vi "Test Set Row Values Append Numbers.vi"(11 "Test Case In":refnum<class "Test Open Xml.lvclass">) -> (0 "error out":errorcluster, 3 "Test Case Out":refnum<class "Test Open Xml.lvclass">)   [LabVIEW 2020, in "Test Open Xml.lvclass"]
uses:
  Test Open Xml.lvclass
  <vilib>/Astemes/LUnit/Test Case.lvclass
  Source/Open Xml.lvlib
  Source/Cell DataType.ctl
panel:
  out "Numeric":dbl
  # "200 - 3.6sec"
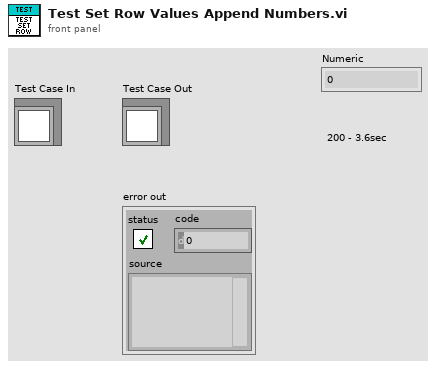
[diagram p1: front panel]
types:
  T1 = typedef "Open Xml.lvlib/Cell DataType.ctl" = enum16{"Void", "Boolean", "Number", "Error", "SharedString", "String", "InlineString", "Date"}
  T2 = cluster{"Number":dbl, "String":string, "Boolean":bool, "Time Stamp":timestamp, "Error":errorcluster}[]
  T3 = cluster{"Number":dbl, "String":string, "Boolean":bool, "Time Stamp":timestamp, "Error":errorcluster}
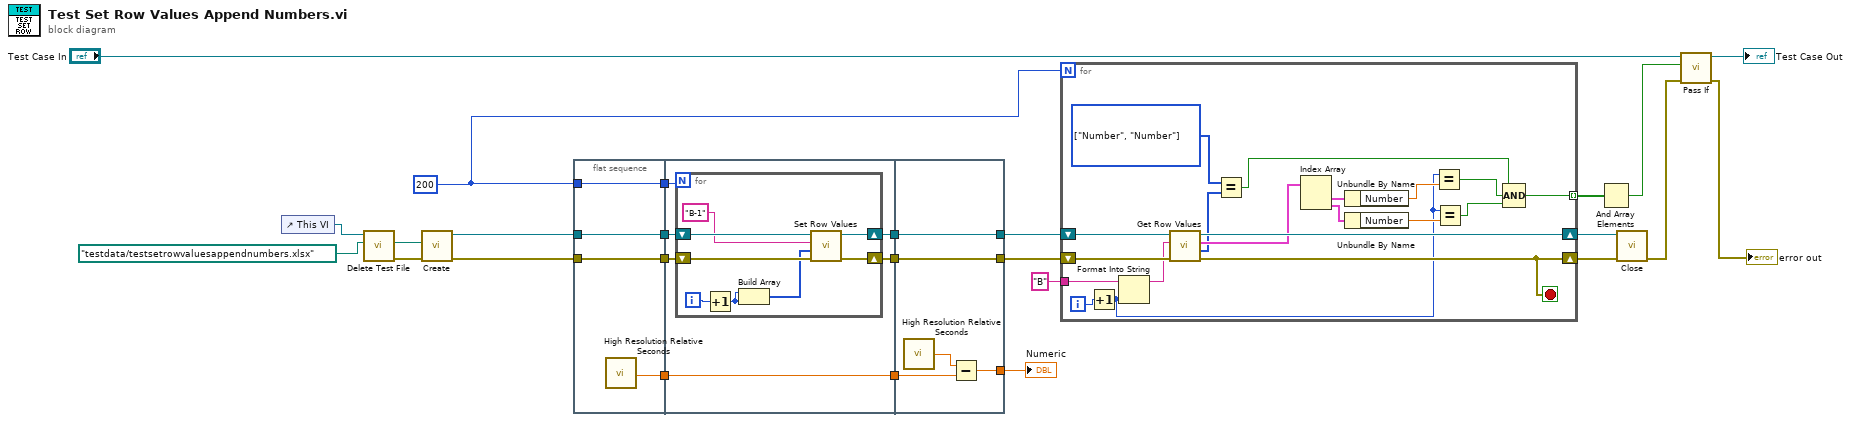
[diagram p0: block diagram]
diagram:
  w11 = 200
  n1 = control-ref of="This VI"() -> (w14:refnum<vi>)
  n2 = call "Delete Test File.vi"("name or relative path"=path "testdata/testsetrowvaluesappendnumbers.xlsx", "VI in"=w14) -> ("error out"=w15:errorcluster, "deleted path"=w12:path)  [unwired: 8 in]
  n3 = call "Create.vi"("error in"=w15, "Path"=w12) -> ("error out"=w22:errorcluster, "SpreadsheetDoc"=w23:refnum<k24>)  [unwired: 8 in]
  n4 = flat-sequence {
    tunnel: w11 -> [w28]
    tunnel: w22 -> [w29]
    tunnel: w23 -> [w30]
    tunnel: [w30] -> w8
    tunnel: [w29] -> w7
    tunnel: [w28] -> w6
    tunnel: [w27] -> w3
    tunnel: w8 -> [w36]
    tunnel: w7 -> [w35]
    tunnel: w6 -> [w32]
    tunnel: [w34] -> w5
    tunnel: [w33] -> w4
    tunnel: w3 -> [w31]
    tunnel: [w31] -> w2
    tunnel: [w48] -> w18
    tunnel: [w49] -> w19
    tunnel: w5 -> [w49]
    tunnel: w4 -> [w48]
    tunnel: w2 -> [w46]
    tunnel: [w45] -> w1
    frame #0 {
      n5 = call <vilib>:"High Resolution Relative Seconds.vi"() -> ("relative seconds"=w27:dbl)
    }
    frame #1 {
      n6 = for {
        N: w32 -> [_]
        shift-right: [w41] -> w33
        shift-left: w36 -> [w44]
        shift-right: [w42] -> w34
        shift-left: w35 -> [w43]
        i -> [w39]
        n7 = Increment(x=w39) -> (x+1=w38:i32)
        n8 = Build Array(w38, w38) -> (w37:i32[])
        n9 = call "Set Row Values.vi"("error in"=w43, "Values"=w37, "Cell Address"="B-1", "SpreadsheetDoc"=w44) -> ("error out"=w42:errorcluster, "SpreadsheetDoc out"=w41:refnum<k24>)  [unwired: 6 in]
      }
    }
    frame #2 {
      n10 = call <vilib>:"High Resolution Relative Seconds.vi"() -> ("relative seconds"=w47:dbl)
      n11 = Subtract(x=w47, y=w46) -> (x-y=w45:dbl)
    }
  }
  n12 = for {
    N: w11 -> [_]
    tunnel: "B" ("Cell Address") -> [w66]
    shift-right: [w51] -> w20
    shift-left: w19 -> [w68]
    shift-right: [w65] -> w16
    shift-left: w18 -> [w67]
    tunnel: [w52] -> w10 mode=indexing
    i -> [w63]
    stop <- w51 stop-if-true
    w62 = T1[] [enum."Number", enum."Number"] items=["Void", "Boolean", "Number", "Error", "SharedString", "String", "InlineString", "Date"] ("x")
    n13 = Increment(x=w63) -> (x+1=w50:i32)
    n14 = Format Into String(initial string=w66, w50) -> (resulting string=w64:string)  [unwired: 2 in, 1 out]
    n15 = call "Get Row Values.vi"("error in"=w68, "Row Address"=w64, "SpreadsheetDoc in"=w67) -> ("error out"=w51:errorcluster, "Types"=w56:T1[], "Cell Values"=w61:T2, "SpreadsheetDoc out"=w65:refnum<k24>)  [unwired: 5 in]
    n16 = Equal?(x=w62, y=w56) -> (x = y?=w53:bool)
    n17 = Index Array(array=w61) -> (element #1=w60:T3, element #2=w59:T3)  [unwired: 2 in]
    n18 = Unbundle By Name(w60) -> ("Number"=w57:dbl)
    n19 = Unbundle By Name(w59) -> ("Number"=w58:dbl)
    n20 = Equal?(x=w50, y=w57) -> (x = y?=w54:bool)
    n21 = Equal?(x=w50, y=w58) -> (x = y?=w55:bool)
    n22 = Compound Arithmetic op=AND(w53, w54, w55) -> (w52:bool)
  }
  n23 = And Array Elements(Boolean array=w10) -> (logical AND=w9:bool)
  n24 = call "Close.vi"("error in"=w20, "SpreadsheetDoc"=w16) -> ("error out"=w21:errorcluster)  [unwired: 9 in]
  n25 = call <vilib>:"Pass If.vi"("error in (no error)"=w21, "Pass?"=w9, "LUnit Test Case In"="Test Case In") -> ("error out"=→"error out":errorcluster, "LUnit Test Case Out"=→"Test Case Out":refnum<class "Test Open Xml.lvclass">)  [unwired: 7 in]
  "Numeric" <- w1
